vi "AlliGator Histogram Bin Size Definition Dialog.vi"(8 "error in (no error)":errorcluster, 9 "Dialog? (T)":bool=TRUE, 11 "Histogram Options in":T1={"Bin Size"=nan, "Bin Number"=0, "Bin Option"=enum."Bin Number", "Min Value"=nan, "Max Value"=nan, "Filter NaN & Infinite Values"=FALSE, "Frequency Plot"=FALSE, "Align Bins"=FALSE, "Bin Location"=enum."Left", "Project Outside Values"=FALSE, "Max Histogram Size"=-1} {"Max Histogram Size" format="%.0e"}) -> (0 "error out":errorcluster, 1 "Cancelled?":bool, 2 "Intensity-weighted Histogram (out)":bool, 3 "Histogram Options":T1={"Bin Size"=1.0, "Bin Number"=0, "Bin Option"=enum."Bin Number", "Min Value"=1.0, "Max Value"=1.0, "Filter NaN & Infinite Values"=FALSE, "Frequency Plot"=FALSE, "Align Bins"=FALSE, "Bin Location"=enum."Left", "Project Outside Values"=FALSE, "Max Histogram Size"=1} {"Max Histogram Size" format="%.0e"}, 4 "Normalized Weighted Histogram (out)":bool)   [LabVIEW 2021, in "AlliGator Lifetime & Other Parameters.lvlib"]
doc: "Displays a standard dialog box that prompts users to enter information, such as a user name and password.\n--------------------\n\nThis Express VI is configured as follows:\n\nMessage to Display to the User:Histogram bin to use:\nThe inputs are: \nNumber: Bin"
uses:
  AlliGator Lifetime & Other Parameters.lvlib
  Histograms/Linear Histogram Options.ctl
  Histograms/Histogram Bin Option.ctl
  Histograms/Histogram Bin Position.ctl
  Histograms/Histogram Window.lvlib
panel:
  in  "Normalized Weighted Histogram":bool
  in  "Intensity-weighted Histogram":bool
  in  "Histogram Options 2":T1={"Bin Size"=1.0, "Bin Number"=100, "Bin Option"=enum."Bin Number", "Min Value"=nan, "Max Value"=nan, "Filter NaN & Infinite Values"=TRUE, "Frequency Plot"=FALSE, "Align Bins"=FALSE, "Bin Location"=enum."Left", "Project Outside Values"=FALSE, "Max Histogram Size"=100000} caption="Histogram Options" {"Max Histogram Size" format="%.0e"}
  in  "Cancel":bool
  in  "OK":bool caption="OK1"
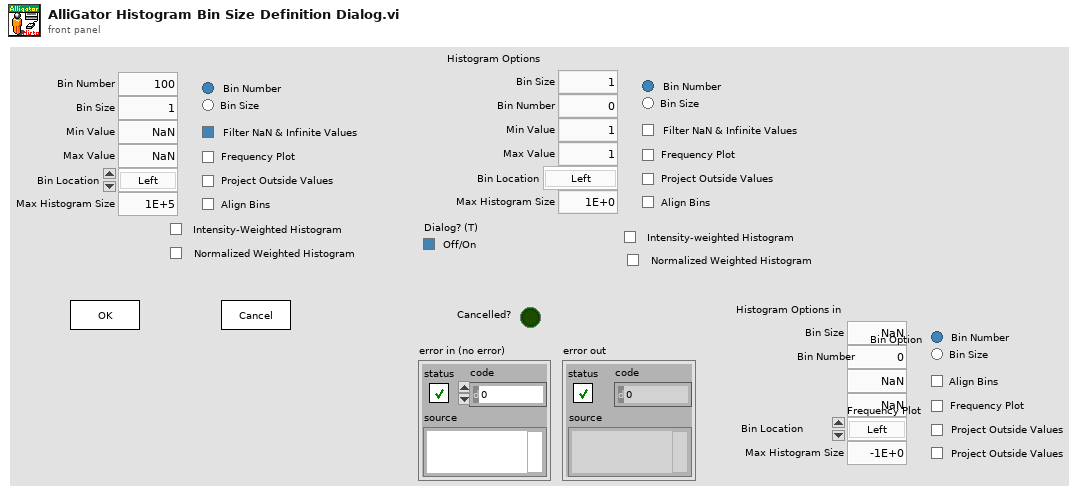
[diagram p1: front panel]
types:
  T1 = typedef "Histogram Window.lvlib/Linear Histogram Options.ctl" = cluster{"Bin Size":dbl, "Bin Number":i32, "Bin Option":T2, "Min Value":dbl, "Max Value":dbl, "Filter NaN & Infinite Values":bool, "Frequency Plot":bool, "Align Bins":bool, "Bin Location":T3, "Project Outside Values":bool, "Max Histogram Size":i32}
  T2 = typedef "Histogram Window.lvlib/Histogram Bin Option.ctl" = enum32{"Bin Number", "Bin Size"}
  T3 = typedef "Histogram Window.lvlib/Histogram Bin Position.ctl" = enum16{"Left", "Center", "Right"}
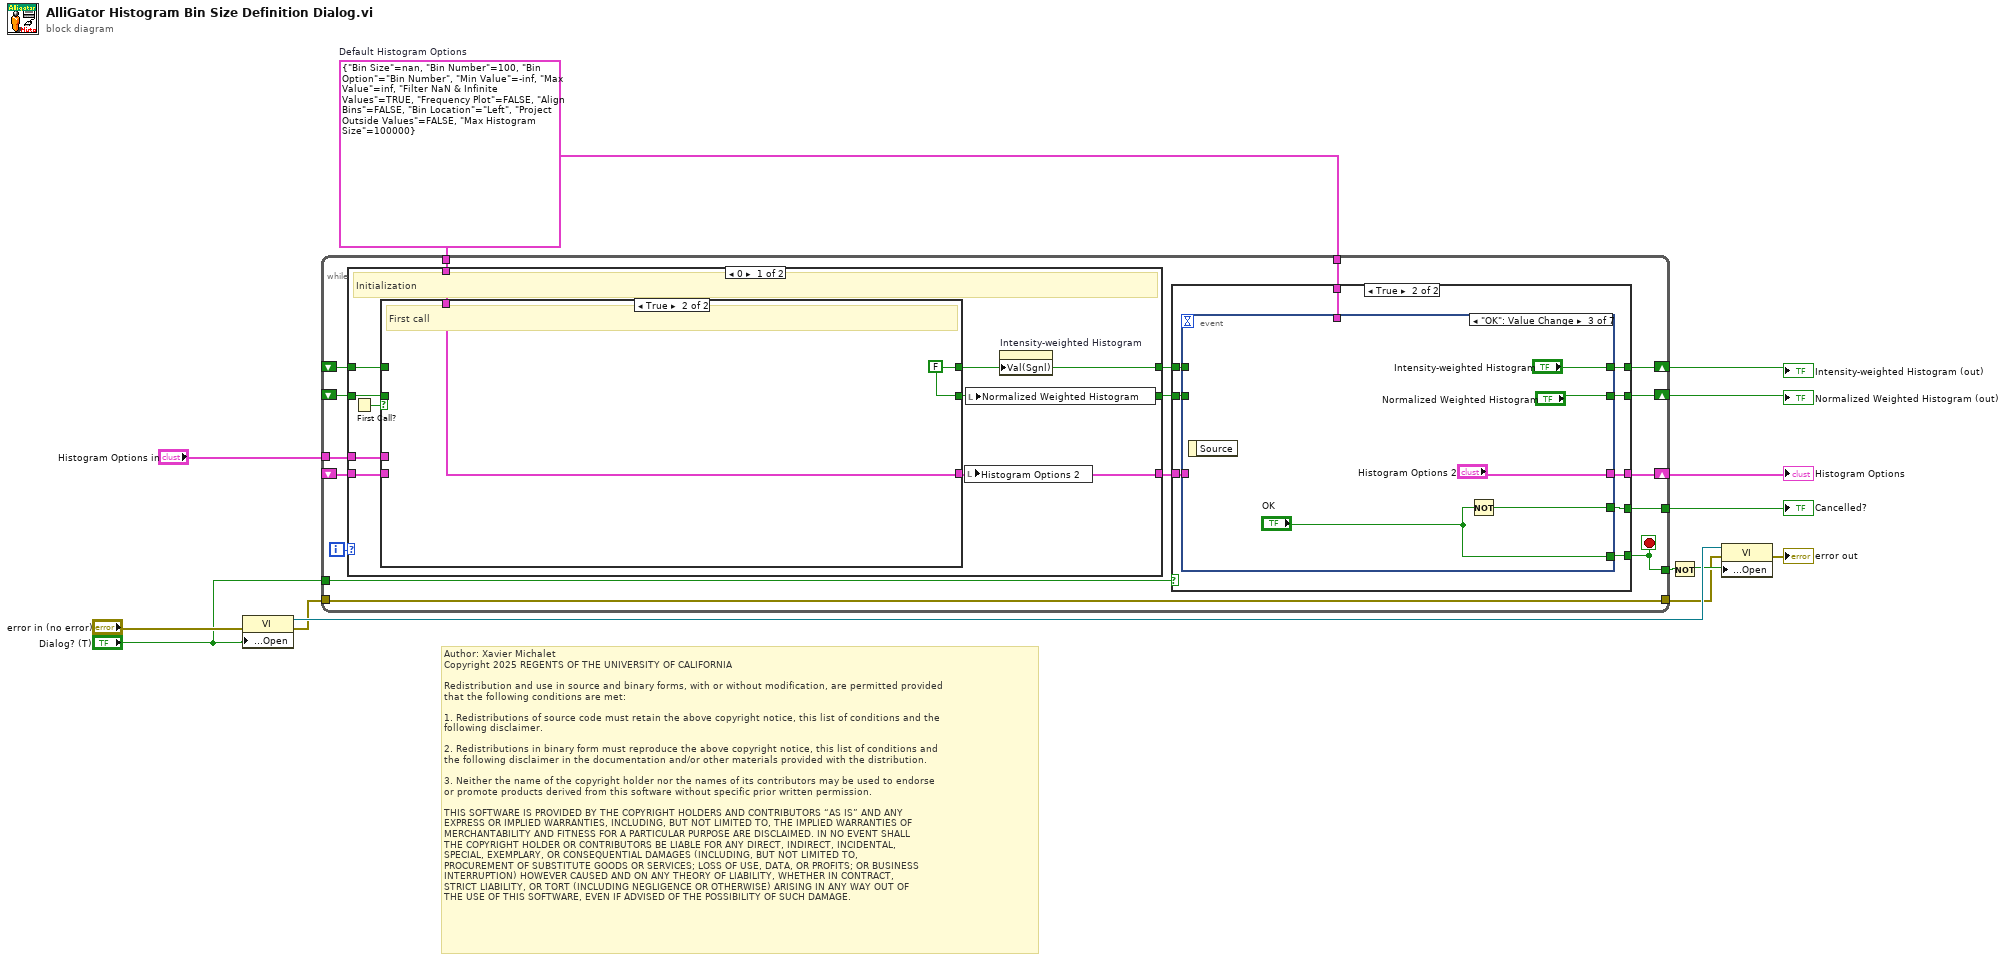
[diagram p0: block diagram]
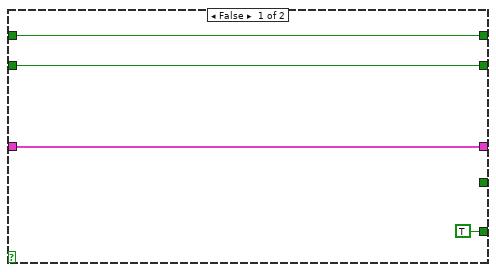
[diagram p2: hidden frame]
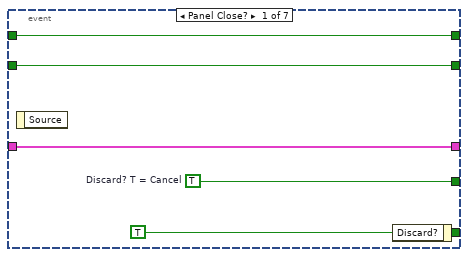
[diagram p3: hidden frame]
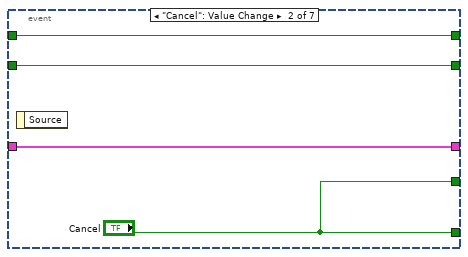
[diagram p4: hidden frame]
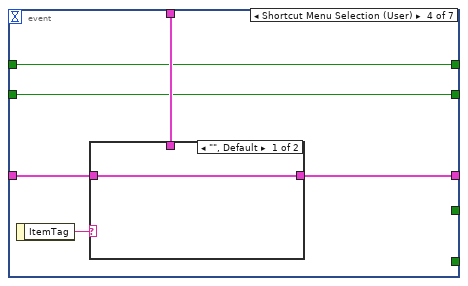
[diagram p5: hidden frame]
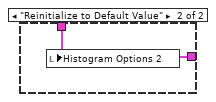
[diagram p6: hidden frame]
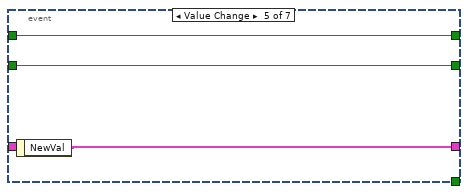
[diagram p7: hidden frame]
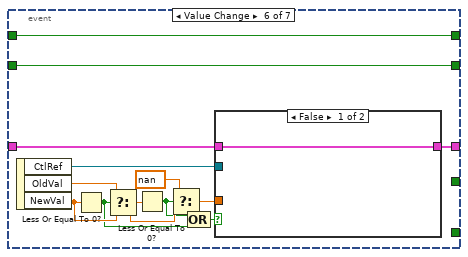
[diagram p8: hidden frame]
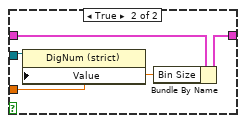
[diagram p9: hidden frame]
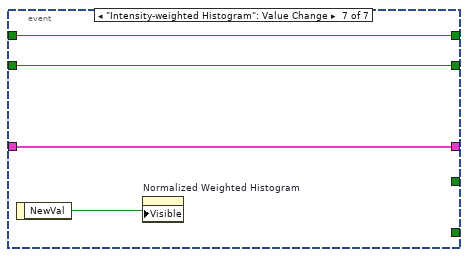
[diagram p10: hidden frame]
diagram:
  w7 = T1 {"Bin Size"=nan, "Bin Number"=100, "Bin Option"=enum."Bin Number", "Min Value"=-inf, "Max Value"=inf, "Filter NaN & Infinite Values"=TRUE, "Frequency Plot"=FALSE, "Align Bins"=FALSE, "Bin Location"=enum."Left", "Project Outside Values"=FALSE, "Max Histogram Size"=100000}  # Default Histogram Options
  # "Author: Xavier Michalet\nCopyright 2025 REGENTS OF THE UNIVERSITY OF CALIFORNIA\n\nRedistribution and use in source and binary forms, with or without modification, are permitted provided\nthat the following conditions are met:\n\n1. Redistributions of source code must retain the above copyright notice, this list of conditions and the\nfollowing disclaimer.\n\n2. Redistributions in binary form must reproduce the above copyright notice, this list of conditions and\nthe following disclaimer in the documentation and/or other materials provided with the distribution.\n\n3. Neither the name of the copyright holder nor the names of its contributors may be used to endorse \nor promote products derived from this software without specific prior written permission.\n\nTHIS SOFTWARE IS PROVIDED BY THE COPYRIGHT HOLDERS AND CONTRIBUTORS “AS IS” AND ANY \nEXPRESS OR IMPLIED WARRANTIES, INCLUDING, BUT NOT LIMITED TO, THE IMPLIED WARRANTIES OF\nMERCHANTABILITY AND FITNESS FOR A PARTICULAR PURPOSE ARE DISCLAIMED. IN NO EVENT SHALL\nTHE COPYRIGHT HOLDER OR CONTRIBUTORS BE LIABLE FOR ANY DIRECT, INDIRECT, INCIDENTAL, \nSPECIAL, EXEMPLARY, OR CONSEQUENTIAL DAMAGES (INCLUDING, BUT NOT LIMITED TO, \nPROCUREMENT OF SUBSTITUTE GOODS OR SERVICES; LOSS OF USE, DATA, OR PROFITS; OR BUSINESS\nINTERRUPTION) HOWEVER CAUSED AND ON ANY THEORY OF LIABILITY, WHETHER IN CONTRACT, \nSTRICT LIABILITY, OR TORT (INCLUDING NEGLIGENCE OR OTHERWISE) ARISING IN ANY WAY OUT OF\nTHE USE OF THIS SOFTWARE, EVEN IF ADVISED OF THE POSSIBILITY OF SUCH DAMAGE."
  n1 = property class="VI"(error in="error in (no error)", "Front Panel Window:Open"="Dialog? (T)") -> (reference out=w11:refnum<vi>, error out=w6:errorcluster)  [unwired: 1 in]
  n2 = while {
    tunnel: [w31] -> w12
    tunnel: [w30] -> w10
    shift-right: [w29] -> w8
    shift-left: _ -> [w27]
    tunnel: w7 -> [w25]
    tunnel: w7 -> [w24]
    tunnel: "Histogram Options in" -> [w23]
    tunnel: w6 -> [w22]
    tunnel: [w22] -> w5
    tunnel: "Dialog? (T)" -> [w21]
    shift-right: [w18] -> w2
    shift-left: _ -> [w20]
    shift-right: [w15] -> w1
    shift-left: _ -> [w17]
    i -> [w28]
    stop <- w30 stop-if-true
    n3 = case "Initialization" shown="0" w28 {
      tunnel: w27 -> [w97 w108]
      tunnel: [w100 w108] -> w26
      tunnel: w25 -> [w96 _]
      tunnel: w23 -> [w99 _]
      tunnel: w20 -> [w95 w107]
      tunnel: [w92 w107] -> w19
      tunnel: w17 -> [w94 w106]
      tunnel: [w93 w106] -> w16
      frame 0 {
        # "Initialization"
        n4 = First Call?() -> (First Call?: T/F=w98:bool)
        n5 = case shown="True" w98 {
          tunnel: [w103 w105] -> w100
          tunnel: w99 -> [_ _]
          tunnel: w97 -> [w103 _]
          tunnel: w96 -> [_ w105]
          tunnel: w95 -> [w102 _]
          tunnel: [w102 w104] -> w92
          tunnel: [w101 w104] -> w93
          tunnel: w94 -> [w101 _]
          frame False {
            # "Not first call: use previous values unless some valid options are provided"
          }
          frame True {
            w104 = FALSE ("Intensity-weighted Histogram")
            # "First call"
          }
        }
        n6 = local write "Histogram Options 2"(w100) -> ()
        n7 = local write "Normalized Weighted Histogram"(w93) -> ()
        n8 = property on="Intensity-weighted Histogram" class="Bool (strict)"("Val(Sgnl)"=w92) -> ()  [unwired: 2 in, 2 out]
      }
      frame 1, Default {
        # "user interaction"
      }
    }
    n9 = case shown="True" w21 {
      tunnel: [_ w44] -> w31
      tunnel: [TRUE ("OK") w43] -> w30
      tunnel: [w35 w42] -> w29
      tunnel: w26 -> [w35 w41]
      tunnel: w24 -> [_ w40]
      tunnel: w19 -> [w33 w39]
      tunnel: [w33 w38] -> w18
      tunnel: w16 -> [w32 w37]
      tunnel: [w32 w36] -> w15
      frame False {
      }
      frame True {
        n10 = event shown="[2] \"OK\": Value Change" {
          selector: _ -> [_ _ _ _ _ _ _]
          dyn-events: _ -> [_ _ _ _ _ _ _]
          timeout: _ -> [_ _ _ _ _ _ _]
          tunnel: [w49 "Cancel" "OK" _ _ _ _] -> w43
          tunnel: [w48 "Cancel" w56 _ _ _ _] -> w44
          tunnel: [w47 w53 "Histogram Options 2" w62 w69 w72 w88] -> w42
          tunnel: w41 -> [w47 w53 _ w63 _ w73 w88]
          tunnel: w40 -> [_ _ _ w61 _ _ _]
          tunnel: w39 -> [w46 w51 _ w60 w68 w71 w89]
          tunnel: [w46 w51 "Intensity-weighted Histogram" w60 w68 w71 w89] -> w38
          tunnel: w37 -> [w45 w50 _ w59 w67 w70 w91]
          tunnel: [w45 w50 "Normalized Weighted Histogram" w59 w67 w70 w91] -> w36
          event Panel Close? {
            w48 = TRUE  # Discard? T = Cancel
            w49 = TRUE ("Discard?")
            n11 = event-data() -> ()  [unwired: 1 in, 1 out]
            n12 = event-data("Discard?"=w49) -> ()  [unwired: 1 in, 1 out]
          }
          event "Cancel": Value Change {
            n13 = event-data() -> ()  [unwired: 1 in, 1 out]
          }
          event "OK": Value Change {
            n14 = event-data() -> ()  [unwired: 1 in, 1 out]
            n15 = Not(x="OK") -> (.not. x?=w56:bool)
          }
          event Shortcut Menu Selection (User) {
            n16 = event-data() -> ("ItemTag"=w64:string)  [unwired: 1 in]
            n17 = case shown="\"\", Default" w64 {
              tunnel: w63 -> [w65 _]
              tunnel: [w65 w66] -> w62
              tunnel: w61 -> [_ w66]
              frame "", Default {
              }
              frame "Reinitialize to Default Value" {
                n18 = local write "Histogram Options 2"(w66) -> ()
              }
            }
          }
          event Value Change {
            n19 = event-data() -> ("NewVal"=w69:T1)  [unwired: 1 in]
          }
          event Value Change {
            n20 = event-data() -> ("CtlRef"=w75:refnum<vi>, "OldVal"=w81:dbl, "NewVal"=w82:dbl)  [unwired: 1 in]
            n21 = Less Or Equal To 0?(x=w82) -> (x <= 0?=w76:bool)
            n22 = Select(t=w81, s=w76, f=w82) -> (s? t:f=w80:dbl)
            n23 = Less Or Equal To 0?(x=w80) -> (x <= 0?=w78:bool)
            n24 = Select(t=nan, s=w78, f=w80) -> (s? t:f=w74:dbl)
            n25 = Compound Arithmetic op=OR(w78, w76) -> (w77:bool)
            n26 = case shown="False" w77 {
              tunnel: w75 -> [_ w87]
              tunnel: w74 -> [_ w85]
              tunnel: w73 -> [w83 w86]
              tunnel: [w83 w84] -> w72
              frame False {
              }
              frame True {
                n27 = property class="DigNum (strict)"(reference=w87, "Value"=w85) -> ()  [unwired: 1 in, 2 out]
                n28 = Bundle By Name(cluster=w86, "Bin Size"=w85) -> (w84:T1)
              }
            }
          }
          event "Intensity-weighted Histogram": Value Change {
            n29 = event-data() -> ("NewVal"=w90:bool)  [unwired: 1 in]
            n30 = property on="Normalized Weighted Histogram" class="Bool (strict)"("Visible"=w90) -> ()  [unwired: 2 in, 2 out]
          }
        }
      }
    }
  }
  "Cancelled?" <- w12
  "Histogram Options" <- w8
  "Intensity-weighted Histogram (out)" <- w2
  "Normalized Weighted Histogram (out)" <- w1
  n31 = Not(x=w10) -> (.not. x?=w9:bool)
  n32 = property class="VI"(reference=w11, error in=w5, "Front Panel Window:Open"=w9) -> (error out=→"error out":errorcluster)  [unwired: 1 out]
